vi "EH Safe Mode Filter.vi"(0 "Father of all uServices in":refnum<class "Father of all uServices.lvclass">, 5 "Event type":T1=enum."Message", 7 "Item Name":string, 9 "Data":variant, 11 "error in (no error)":errorcluster) -> (4 "Father of all uServices out":refnum<class "Father of all uServices.lvclass">, 6 "Event type out":T1=enum."Message", 8 "Item Name out":string, 10 "Data out":variant, 14 "Execute":bool, 15 "error out":errorcluster)   [LabVIEW 2026, in "TALOS.lvlib" / "Father of all uServices.lvlib" / "Father of all uServices.lvclass"]
uses:
  Father of all uServices.lvclass
  Event Handler Items.ctl
  e9a4b515-168a-4185-aa25-a46393002024.vi
  <vilib>/AdvancedString/Delimited String to 1D String Array.vi
  <vilib>/AdvancedString/Delimited String to 1D String Array (string).vi
  Support VIs/Global Constants.vi
  <vilib>/Utility/LVClass/Get LV Class Name.vi
  <vilib>/Comparison/Equal/Equal Functor/Equal Functor.lvclass
  TALOS.lvlib
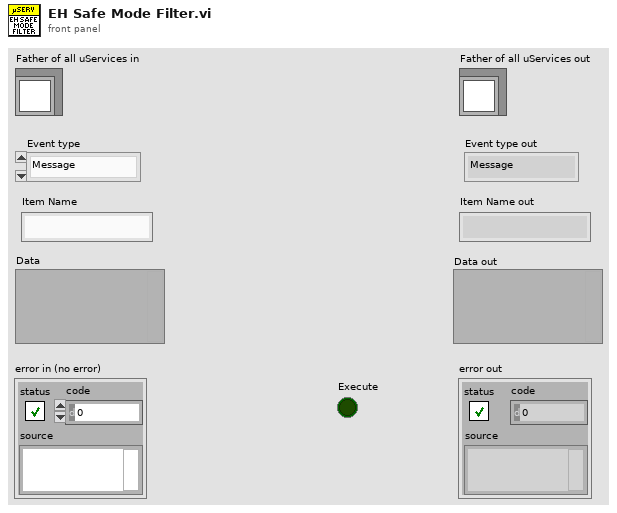
[diagram p1: front panel]
types:
  T1 = typedef "TALOS.lvlib/Father of all uServices.lvlib/Father of all uServices.lvclass/Event Handler Items.ctl" = enum16{"Button Pressed", "Message", "Ready to launch?", "Safe Mode", "Start RUN", "Stop RUN"}
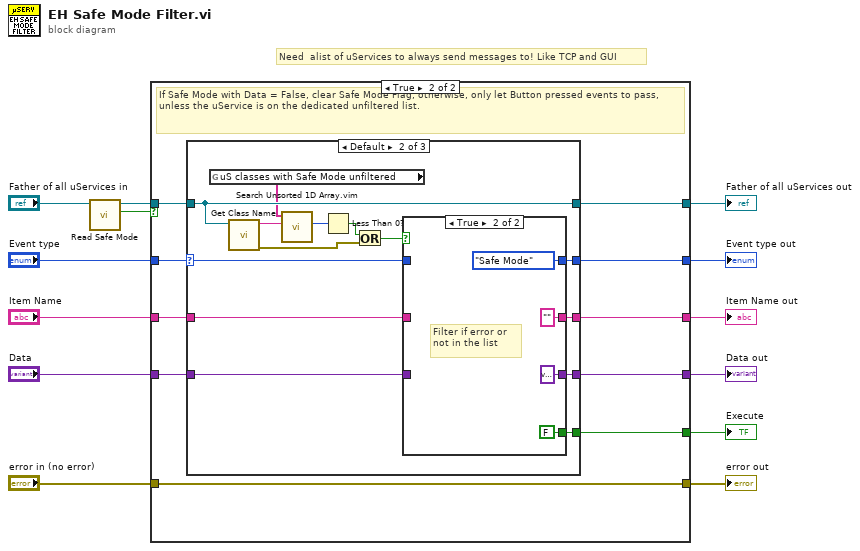
[diagram p0: block diagram]
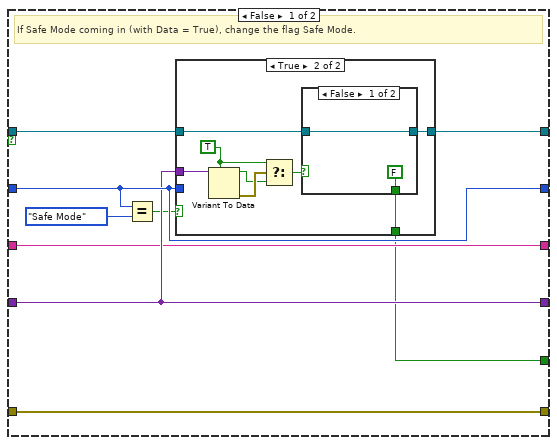
[diagram p2: hidden frame]
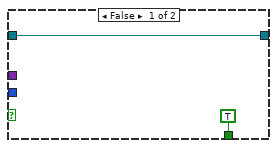
[diagram p3: hidden frame]
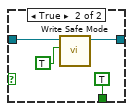
[diagram p4: hidden frame]
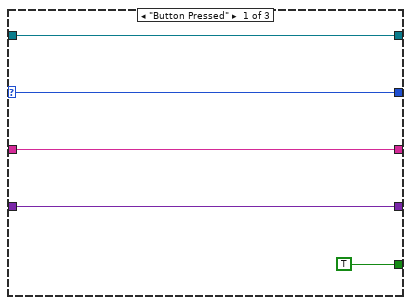
[diagram p5: hidden frame]
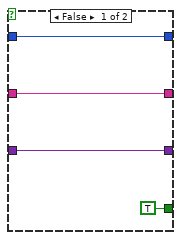
[diagram p6: hidden frame]
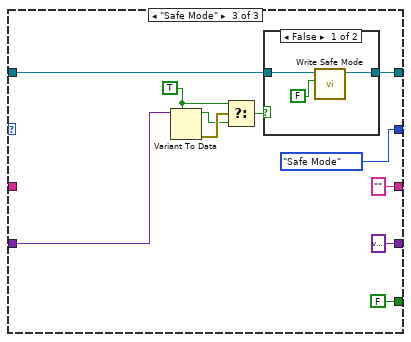
[diagram p7: hidden frame]
diagram:
  # "Need  alist of uServices to always send messages to! Like TCP and GUI"
  n1 = call-dynamic "Read Safe Mode.vi"("Ancestor in"="Father of all uServices in") -> ("Safe Mode"=w5:bool, "Ancestor out"=w6:refnum<class "Father of all uServices.lvclass">)  [unwired: 8 in, 1 out]
  n2 = case shown="True" w5 {
    tunnel: "error in (no error)" -> [w16 w48]
    tunnel: [w16 w48] -> w12
    tunnel: w6 -> [w18 w47]
    tunnel: "Event type" -> [w22 w44]
    tunnel: "Item Name" -> [w15 w42]
    tunnel: "Data" -> [w21 w45]
    tunnel: [w19 w46] -> w8
    tunnel: [w22 w43] -> w4
    tunnel: [w21 w40] -> w3
    tunnel: [w14 w39] -> w2
    tunnel: [w15 w41] -> w1
    frame False {
      # "If Safe Mode coming in (with Data = True), change the flag Safe Mode."
      n3 = Equal?(x=w22, y=Event_Handler_Items."Safe Mode" ("Event type")) -> (x = y?=w17:bool)
      n4 = case shown="True" w17 {
        tunnel: [w24 w32] -> w19
        tunnel: w18 -> [w24 w31]
        tunnel: w22 -> [_ _]
        tunnel: w21 -> [_ w30]
        tunnel: [TRUE w25] -> w14
        frame False {
        }
        frame True {
          w27 = TRUE
          n5 = Variant To Data(type=w27, Variant=w30) -> (data=w28:bool, error out=w29:errorcluster)  [unwired: 1 in]
          n6 = Select(t=w27, s=w29, f=w28) -> (s? t:f=w26:bool)
          n7 = case shown="False" w26 {
            tunnel: [w34 w38] -> w32
            tunnel: w31 -> [w34 w37]
            tunnel: [FALSE TRUE] -> w25
            frame False {
            }
            frame True {
              n8 = call-dynamic "Write Safe Mode.vi"("Safe Mode"=TRUE, "Ancestor in"=w37) -> ("Ancestor out"=w38:refnum<class "Father of all uServices.lvclass">)  [unwired: 8 in, 1 out]
            }
          }
        }
      }
    }
    frame True {
      # "If Safe Mode with Data = False, clear Safe Mode Flag; otherwise, only let Button pressed events to pass, unless the uService is on the dedicated unfiltered list."
      n9 = case shown="Default" w44 {
        selector: w44 -> [w52 w62 _]
        tunnel: w47 -> [w53 w63 w82]
        tunnel: [w53 w63 w81] -> w46
        tunnel: w45 -> [w50 w60 w80]
        tunnel: [w52 w64 Event_Handler_Items."Safe Mode" ("Event type")] -> w43
        tunnel: w42 -> [w51 w61 _]
        tunnel: [w51 w65 "" ("Item Name")] -> w41
        tunnel: [w50 w66 variant ("Data")] -> w40
        tunnel: [TRUE w67 FALSE] -> w39
        frame "Button Pressed" {
        }
        frame Default {
          n10 = global read "Global Constants.vi" "uS classes with Safe Mode unfiltered"() -> (w59:string[])
          n11 = call "Get Class Name.vi"("object"=w63) -> ("error out"=w55:errorcluster, "Class Name"=w58:string)  [unwired: 9 in]
          n12 = call "Search Unsorted 1D Array.vim"("element"=w58, "unsorted 1D array"=w59) -> ("index of element"=w57:i32)  [unwired: 9 in]
          n13 = Less Than 0?(x=w57) -> (x < 0?=w56:bool)
          n14 = Or(x=w56, y=w55) -> (x .or. y?=w54:bool)
          n15 = case shown="True" w54 {
            tunnel: [TRUE FALSE] -> w67
            tunnel: [w69 variant ("Data")] -> w66
            tunnel: [w70 "" ("Item Name")] -> w65
            tunnel: [w71 Event_Handler_Items."Safe Mode" ("Event type")] -> w64
            tunnel: w62 -> [w71 _]
            tunnel: w61 -> [w70 _]
            tunnel: w60 -> [w69 _]
            frame False {
            }
            frame True {
              # "Filter if error or not in the list"
            }
          }
        }
        frame "Safe Mode" {
          w84 = TRUE
          n16 = Variant To Data(type=w84, Variant=w80) -> (data=w85:bool, error out=w86:errorcluster)  [unwired: 1 in]
          n17 = Select(t=w84, s=w86, f=w85) -> (s? t:f=w83:bool)
          n18 = case shown="False" w83 {
            tunnel: [w89 w90] -> w81
            tunnel: w82 -> [w88 w90]
            frame False {
              n19 = call-dynamic "Write Safe Mode.vi"("Safe Mode"=FALSE, "Ancestor in"=w88) -> ("Ancestor out"=w89:refnum<class "Father of all uServices.lvclass">)  [unwired: 8 in, 1 out]
            }
            frame True {
            }
          }
        }
      }
    }
  }
  "error out" <- w12
  "Father of all uServices out" <- w8
  "Execute" <- w2
  "Event type out" <- w4
  "Data out" <- w3
  "Item Name out" <- w1
